vi "get_counter.vi"(8 "error in (no error)":errorcluster, 11 "SignalWriterDL090202DAQmx in":refnum<class "SignalWriterDL090202DAQmx.lvclass">) -> (0 "error out":errorcluster, 1 "not empty?":bool, 2 "counter":tag, 3 "SignalWriterDL090202DAQmx out":refnum<class "SignalWriterDL090202DAQmx.lvclass">)   [LabVIEW 2010, in "SignalWriterDL090202DAQmx.lvclass"]
uses:
  SignalWriterDL090202DAQmx.lvclass
  SignalWriterDL090202DAQmx.lvclass/SignalWriterDL090202DAQmx.ctl
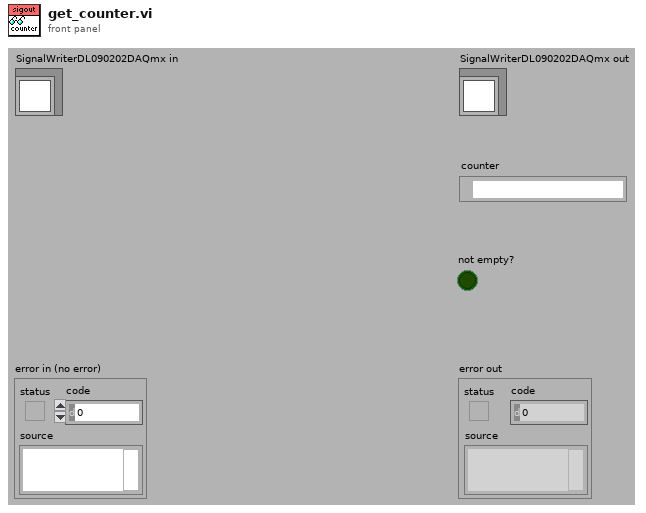
[diagram p1: front panel]
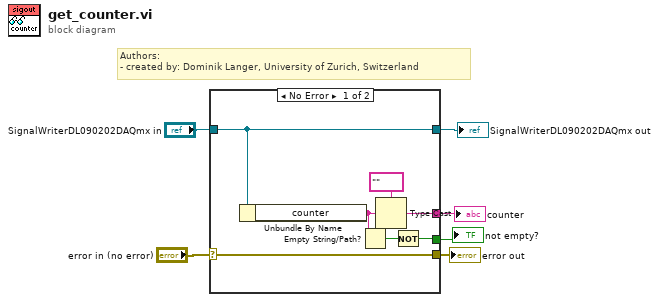
[diagram p0: block diagram]
diagram:
  # "Authors: \n- created by: Dominik Langer, University of Zurich, Switzerland"
  n1 = case shown="No Error" "error in (no error)" {
    selector: "error in (no error)" -> [w13 w15]
    tunnel: [w13 w15] -> w5
    tunnel: [w12 w14] -> w3
    tunnel: "SignalWriterDL090202DAQmx in" -> [w12 w14]
    tunnel: [w11 _] -> w2
    tunnel: [w7 _] -> w1
    frame No Error {
      n2 = Unbundle By Name(w12) -> ("counter"=w9:string)
      n3 = Empty String/Path?(string/path=w9) -> (empty?=w8:bool)
      n4 = Type Cast(type=tag "" ("counter"), x=w9) -> (*(type *) &x=w11:tag)
      n5 = Not(x=w8) -> (.not. x?=w7:bool)
    }
    frame Error {
    }
  }
  "error out" <- w5
  "SignalWriterDL090202DAQmx out" <- w3
  "counter" <- w2
  "not empty?" <- w1
